vi "Lights Teleop.vi"   [LabVIEW 2023]
uses:
  source files/Amp-Speaker.ctl
  source files/Lights Setpoints.ctl
  Implementation/LED Operations.ctl
  Framework/Robot Global Data.vi
types:
  T1 = typedef "LED Operations.ctl" = enum16{"Reserve", "Read Current", "Immediate"}
  T2 = typedef "Lights Setpoints.ctl" = enum16{"Speaker", "Amp"}
  T3 = typedef "Amp-Speaker.ctl" = enum16{"Default", "Flywheel State", "Endgame", "Note Detection"}
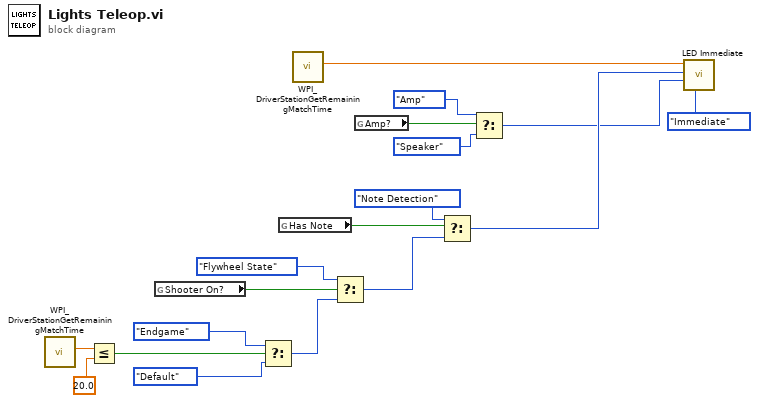
[diagram p0: block diagram]
diagram:
  n1 = call <vilib>:"WPI_DriverStationGetRemainingMatchTime.vi"() -> ("Match Time(s)"=w8:sgl)  [unwired: 10 in, 1 out]
  n2 = Less Or Equal?(x=w8, y=sgl 20.0) -> (x <= y?=w6:bool)
  n3 = global read "Robot Global Data.vi" "Shooter On?"() -> (w10:bool)
  n4 = Select(t=Amp-Speaker."Endgame" ("Lights State"), s=w6, f=Amp-Speaker."Default" ("Lights State")) -> (s? t:f=w14:T3)
  n5 = global read "Robot Global Data.vi" "Has Note"() -> (w11:bool)
  n6 = call <vilib>:"WPI_DriverStationGetRemainingMatchTime.vi"() -> ("Match Time(s)"=w18:sgl)  [unwired: 10 in, 1 out]
  n7 = Select(t=Amp-Speaker."Flywheel State" ("Lights State"), s=w10, f=w14) -> (s? t:f=w16:T3)
  n8 = global read "Robot Global Data.vi" "Amp?"() -> (w5:bool)
  n9 = Select(t=Amp-Speaker."Note Detection" ("Lights State"), s=w11, f=w16) -> (s? t:f=w12:T3)
  n10 = Select(t=Lights_Setpoints."Amp" ("Amp or Speaker"), s=w5, f=Lights_Setpoints."Speaker" ("Amp or Speaker")) -> (s? t:f=w2:T2)
  n11 = call "LED Immediate.vi"("Operation"=LED_Operations."Immediate", "Amp or Speaker"=w2, "Lights State"=w12, "Match Time"=w18) -> ()  [unwired: 7 in, 1 out]
